vi "Chat Launcher.vi"() -> ()   [LabVIEW 2020, in "Simple Chat.lvlib"]
uses:
  Simple Chat.lvlib
  Simple Chat/Simple Chat.lvclass
  <vilib>/ActorFramework/Actor/Actor.lvclass
  <vilib>/ActorFramework/Stop Msg/Stop Msg.lvclass
  Actor Pub Sub Channels/Actor Pub Sub Channels.lvlib
  Actor Pub Sub Channels/Helpers/Get Topic Enqueuer.vi
  Actor Pub Sub Channels/Pub Sub Retaining Message Channel/Pub Sub Retaining Message Channel.lvclass
  C:/Users/Simon/Documents/GitHub/LV-Actor-Pub-Sub/Source/Actor Pub Sub Channels/Pub Sub Message Channel/Pub Sub Message Channel.lvclass
  C:/Program Files (x86)/National Instruments/LabVIEW 2020/vi.lib/ActorFramework/Actor/Actor.lvclass
panel:
  in  "stop":bool
  in  "Start Actor":bool
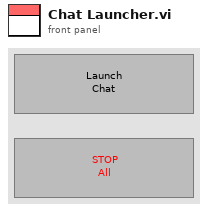
[diagram p1: front panel]
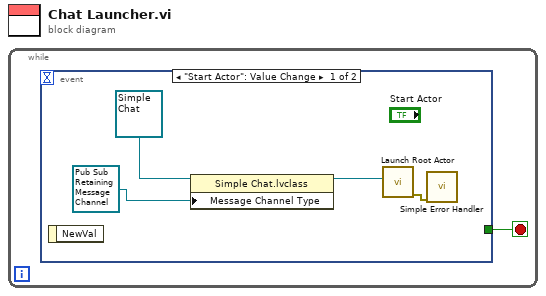
[diagram p0: block diagram]
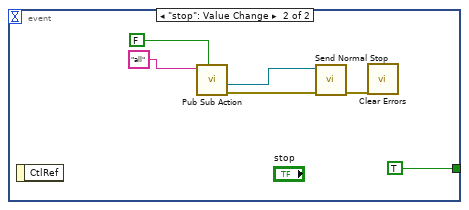
[diagram p2: hidden frame]
diagram:
  n1 = while {
    stop <- w1 stop-if-true
    n2 = event shown="[0] \"Start Actor\": Value Change" {
      selector: _ -> [_ _]
      dyn-events: _ -> [_ _]
      timeout: _ -> [_ _]
      tunnel: [_ TRUE] -> w1
      event "Start Actor": Value Change {
        n3 = event-data() -> ()  [unwired: 1 in, 1 out]
        n4 = property class="Simple Chat.lvclass"(reference=refnum<class "Simple Chat.lvclass"> refnum ("Simple Chat.lvlib:Simple Chat.lvclass"), "Message Channel Type"=refnum<class "Pub Sub Retaining Message Channel.lvclass"> refnum ("Actor Pub Sub Channels.lvlib:Pub Sub Retaining Message Channel.lvclass")) -> (reference out=w4:refnum<class "Simple Chat.lvclass">)  [unwired: 1 in, 1 out]
        n5 = call <vilib>:"Launch Root Actor.vi"("Actor"=w4) -> ("error out"=w2:errorcluster)  [unwired: 9 in, 1 out]
        n6 = call <vilib>:"Simple Error Handler.vi"("error in (no error)"=w2) -> ()  [unwired: 4 in, 5 out]
      }
      event "stop": Value Change {
        n7 = event-data() -> ()  [unwired: 1 in, 1 out]
        n8 = call-poly "Pub Sub Action.vi"("Create if not exist? (T)"=FALSE, "Topic"="all") -> ("error out"=w9:errorcluster, "Topic Enqueuer"=w10:refnum<class "Message Enqueuer.lvclass">)  [unwired: 6 in, 2 out]
        n9 = call <vilib>:"Send Normal Stop.vi"("error in (no error)"=w9, "Message Enqueuer"=w10) -> ("error out"=w6:errorcluster)  [unwired: 9 in]
        n10 = call <vilib>:"Clear Errors.vi"("error in (no error)"=w6) -> ()  [unwired: 5 in, 2 out]
      }
    }
  }
